vi "eFGV - Stop RT.vi"(6 "State":T1, 8 "Error In":errorcluster, 11 "Stop RT? In":bool) -> (0 "Error Out":errorcluster, 2 "Event Stop RT":refnum<user-event>, 3 "Stop RT? Out":bool)   [LabVIEW 2020]
uses:
  Control/State - eFGV.ctl
  <vilib>/event_ctls.llb/usereventprio.ctl
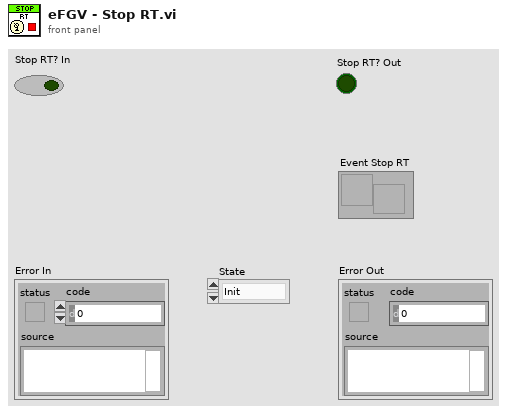
[diagram p1: front panel]
types:
  T1 = typedef "State - eFGV.ctl" = enum16{"Init", "Read", "Write", "Exit"}
  T2 = typedef "usereventprio.ctl" = enum32{"high priority", "normal priority"}
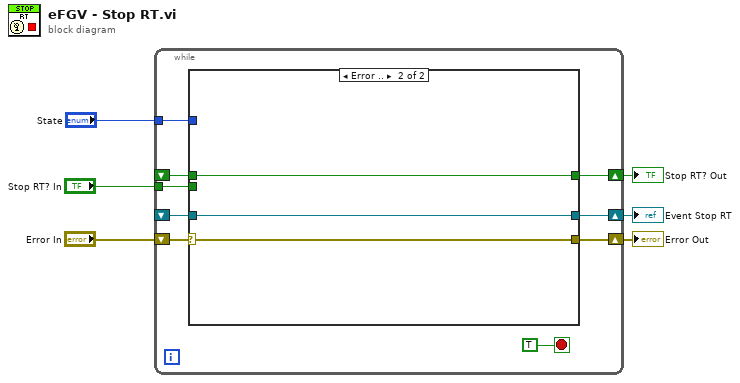
[diagram p0: block diagram]
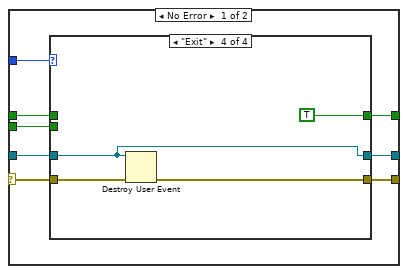
[diagram p2: hidden frame]
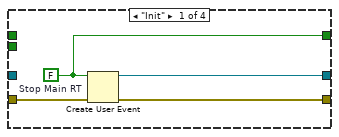
[diagram p3: hidden frame]
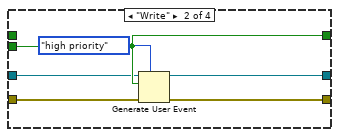
[diagram p4: hidden frame]
diagram:
  n1 = while {
    tunnel: "State" -> [w12]
    shift-right: [w15] -> w6
    shift-left: "Error In" -> [w14]
    tunnel: "Stop RT? In" -> [w11]
    shift-right: [w10] -> w3
    shift-left: _ -> [w9]
    shift-right: [w8] -> w2
    shift-left: _ -> [w7]
    stop <- TRUE stop-if-true
    n2 = case shown="Error .." w14 {
      selector: w14 -> [w22 w43]
      tunnel: [w23 w43] -> w15
      tunnel: w12 -> [w21 _]
      tunnel: w11 -> [w20 _]
      tunnel: [w19 w42] -> w10
      tunnel: w9 -> [w18 w42]
      tunnel: [w17 w41] -> w8
      tunnel: w7 -> [w16 w41]
      frame No Error {
        n3 = case shown="\"Exit\"" w21 {
          tunnel: w22 -> [w27 w33 w36 w40]
          tunnel: [w26 w32 w36 w39] -> w23
          tunnel: w20 -> [_ w31 _ _]
          tunnel: [w25 w31 w35 TRUE ("Stop?")] -> w19
          tunnel: w18 -> [_ _ w35 _]
          tunnel: [w24 w28 w34 w37] -> w17
          tunnel: w16 -> [_ w29 w34 w37]
          frame "Init" {
            w25 = FALSE  # Stop Main RT
            n4 = Create User Event(user event datatype=w25, error in=w27) -> (user event=w24:refnum<user-event>, error out=w26:errorcluster)
          }
          frame "Write" {
            n5 = Generate User Event(priority (normal)=usereventprio."high priority", user event=w29, event data cluster=w31, error in=w33) -> (user event out=w28:refnum<user-event>, error out=w32:errorcluster)
          }
          frame "Read" {
          }
          frame "Exit" {
            n6 = Destroy User Event(user event=w37, error in=w40) -> (error out=w39:errorcluster)
          }
        }
      }
      frame Error {
      }
    }
  }
  "Error Out" <- w6
  "Stop RT? Out" <- w3
  "Event Stop RT" <- w2
